vi "Circuit size update.vi"(11 "Wire in":T1) -> ()   [LabVIEW 2016]
uses:
  TypeDefs/Circuit Cluster.ctl
  Classes/GateAbst/GateAbst.lvclass
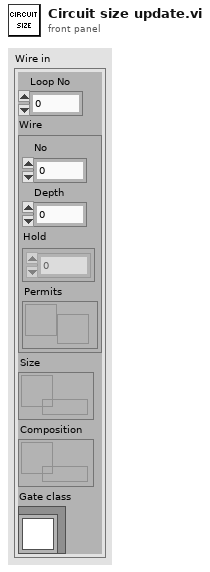
[diagram p1: front panel]
types:
  T1 = typedef "Circuit Cluster.ctl" = cluster{"Loop No":i32, "Wire":cluster{"No":i32, "Depth":i32, "Hold":i32[][], "Permits":refnum<notifier>}, "Size":refnum<queue>, "Composition":refnum<queue>, "Gate class":refnum<class "GateAbst.lvclass">}
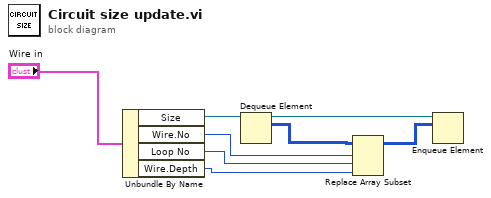
[diagram p0: block diagram]
diagram:
  n1 = Unbundle By Name("Wire in") -> ("Size"=w2:refnum<queue>, "Wire.No"=w5:i32, "Loop No"=w1:i32, "Wire.Depth"=w6:i32)
  n2 = Dequeue Element(queue=w2) -> (queue out=w3:refnum<queue>, element=w4:i32[][])  [unwired: 2 in, 2 out]
  n3 = Replace Array Subset(array=w4, new element=w6, index (row)=w5, index (col)=w1) -> (w7:i32[][])
  n4 = Enqueue Element(queue=w3, element=w7) -> ()  [unwired: 2 in, 3 out]
